vi "Returning Values By Reference Array Of Integers.vi"(7 "newLength":i32, 9 "newArray":i32, 10 "length":i32, 11 "x":i32) -> (1 "newArray out":i32, 3 "x out":i32, 5 "newLength out":i32)   [LabVIEW 2018, in "ParsingDataSampleDLL.lvlib"]
doc: "__declspec(dllexport) void ReturningValuesByReference_ArrayOfIntegers (int *x, int length, int **newArray, int *newLength);"
uses:
  ParsingDataSampleDLL.lvlib
  ni_reference_vs/Debug/ParsingDataSampleDLL.dll
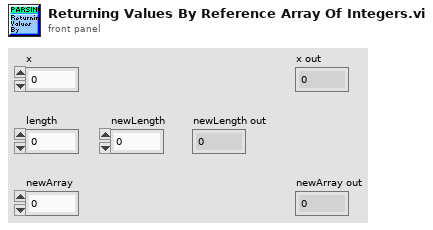
[diagram p1: front panel]
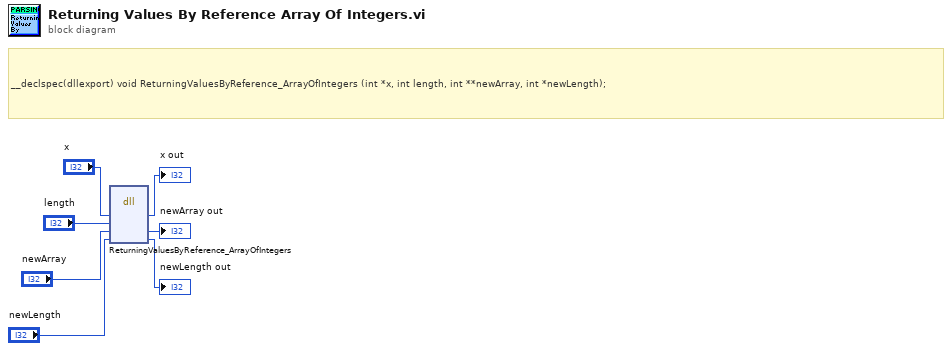
[diagram p0: block diagram]
diagram:
  # "__declspec(dllexport) void ReturningValuesByReference_ArrayOfIntegers (int *x, int length, int **newArray, int *newLength);"
  n1 = dll-call lib="C:/Users/celit/Documents/GitHub/Labview_Python_DLL_Call/ni_reference_vs/Debug/ParsingDataSampleDLL.*" fn="ReturningValuesByReference_ArrayOfIntegers"("x"="x", "length"="length", "newArray"="newArray", "newLength"="newLength") -> ("x"=→"x out":i32, "newArray"=→"newArray out":i32, "newLength"=→"newLength out":i32)  [unwired: 5 in, 2 out]
